vi "Aula 2.vi"() -> ()   [LabVIEW 2024]
panel:
  in  "Boolean":bool
  out "Iterações":dbl
  out "Temperatura ºC":dbl(slide) scale=0.0..100.0
  out "Temperatura ºC":dbl
  in  "Temperatura ºF":dbl(slide) scale=0.0..273.0
  in  "stop":bool
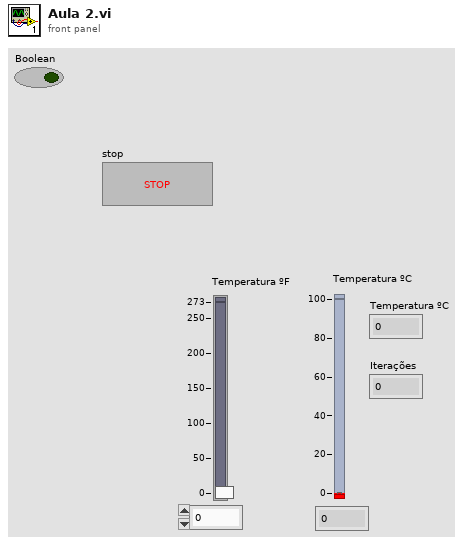
[diagram p1: front panel]
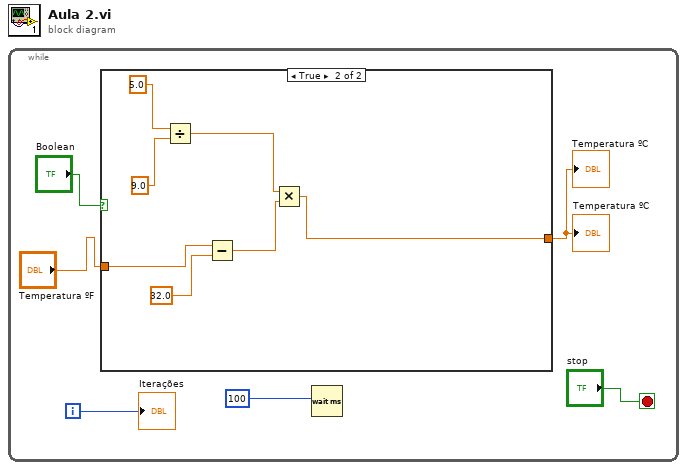
[diagram p0: block diagram]
diagram:
  n1 = while {
    i -> [w6]
    stop <- "stop" stop-if-true
    n2 = case shown="True" "Boolean" {
      tunnel: "Temperatura ºF" -> [w7 w9]
      tunnel: [w7 w8] -> w4
      frame False {
      }
      frame True {
        n3 = Divide(x=5.0, y=9.0) -> (x/y=w11:dbl)
        n4 = Subtract(x=w9, y=32.0) -> (x-y=w10:dbl)
        n5 = Multiply(x=w11, y=w10) -> (x*y=w8:dbl)
      }
    }
    "Temperatura ºC" <- w4
    "Temperatura ºC" <- w4
    n6 = Wait (ms)(milliseconds to wait=u32 100) -> ()  [unwired: 1 out]
    "Iterações" <- w6
  }
